vi "Make sine signal.vi"(0 "sinfreq":dbl, 1 "stimdur":dbl, 2 "nsamp":dbl, 3 "sinamp":dbl, 5 "Output freq (Hz)":dbl, 7 "hicutoff":dbl, 9 "lowcutoff":dbl, 11 "noiseamp":dbl, 12 "beforedur":dbl, 13 "afterdur":dbl) -> (4 "Stimulus out":T2 {"noise freq hi" min=0.0 step=0.5; "noise freq lo" min=0.0 step=0.5; "noiseamp end" min=0.0 step=0.5; "noiseamp start" min=0.0 step=0.5}, 6 "sine wave":dbl[](array[numeric]), 8 "noise":dbl[](array[numeric]), 10 "phases":T1)   [LabVIEW 2013]
uses:
  Stimulus.ctl
  Stimulus type.ctl
  Pulse data.ctl
  Phases.ctl
  <vilib>/Analysis/NI_AALBase.lvlib
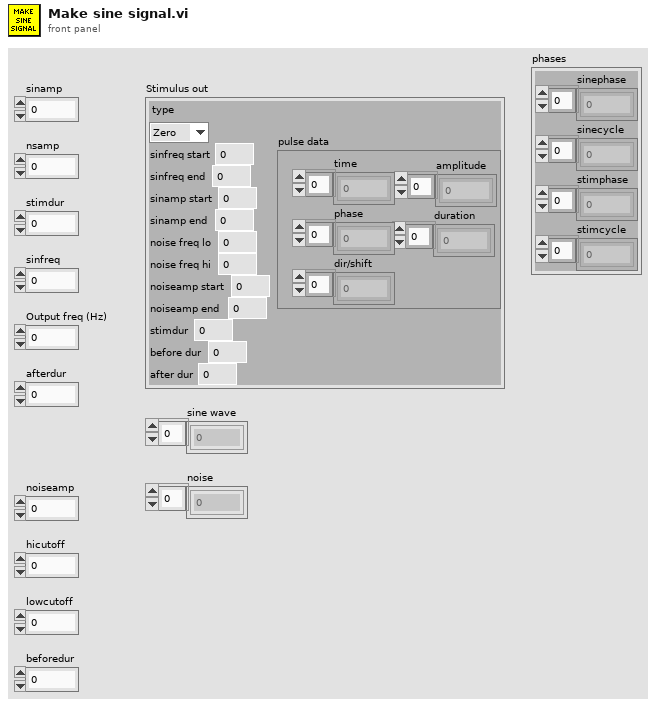
[diagram p1: front panel]
types:
  T1 = typedef "Phases.ctl" = cluster{"sinephase":dbl[], "sinecycle":dbl[], "stimphase":dbl[], "stimcycle":dbl[]}
  T2 = typedef "Stimulus.ctl" = cluster{"type":T3, "sinfreq start":dbl, "sinfreq end":dbl, "sinamp start":dbl, "sinamp end":dbl, "noise freq lo":dbl, "noise freq hi":dbl, "noiseamp start":dbl, "noiseamp end":dbl, "stimdur":dbl, "before dur":dbl, "after dur":dbl, "pulse data":T4}
  T3 = typedef "Stimulus type.ctl" = enum16{"Zero", "Sine", "Frequency sweep", "Two frequency", "Amplitude sweep", "Pulses", "Shifts"}
  T4 = typedef "Pulse data.ctl" = cluster{"time":dbl[], "phase":dbl[], "dir/shift":dbl[], "amplitude":dbl[], "duration":dbl[]}
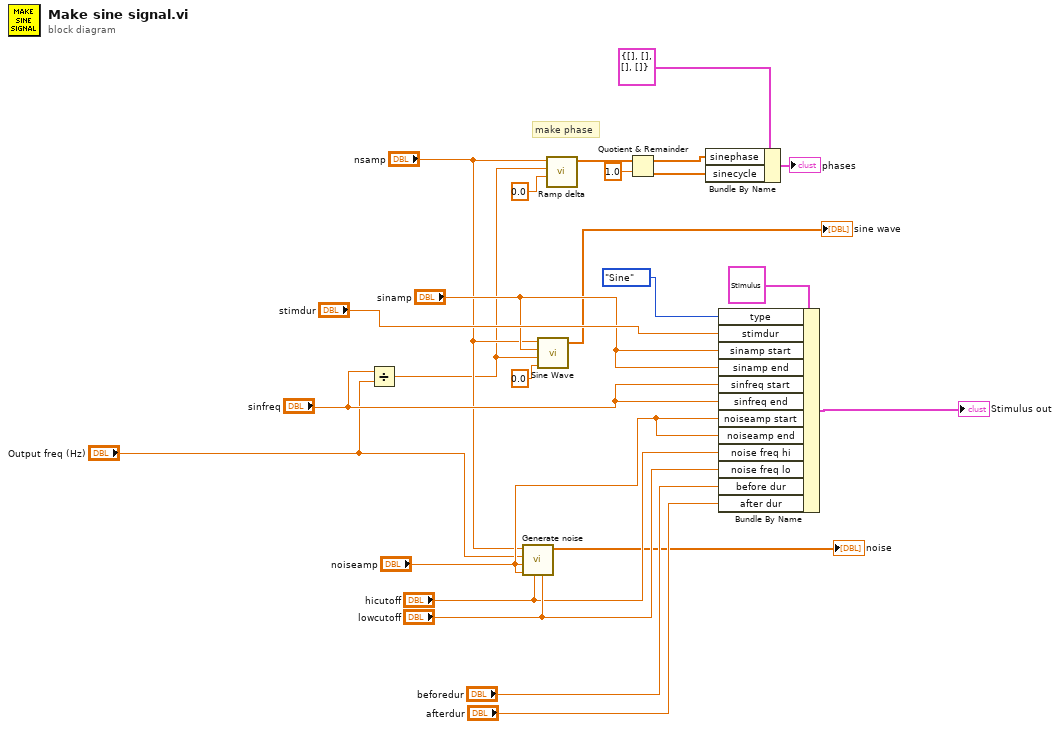
[diagram p0: block diagram]
diagram:
  # "make phase"
  n1 = Divide(x="sinfreq", y="Output freq (Hz)") -> (x/y=w8:dbl)
  n2 = call "Generate noise.vi"("lo cutoff"="lowcutoff", "hi cutoff"="hicutoff", "start amplitude"="noiseamp", "end amplitude"="noiseamp", "sampling freq"="Output freq (Hz)", "samples"="nsamp") -> ("noise"=→"noise":dbl[])  [unwired: 5 in]
  n3 = call <vilib>:"Sine Wave.vi"("samples"="nsamp", "amplitude"="sinamp", "frequency"=w8, "phase in"=0.0) -> ("sine wave"=→"sine wave":dbl[])  [unwired: 1 in, 2 out]
  n4 = call "Ramp delta.vi"("start"=0.0, "delta"=w8, "samples"="nsamp") -> ("ramp signal"=w6:dbl[])  [unwired: 7 in, 1 out]
  n5 = Quotient & Remainder(x=w6, y=1.0 ("start")) -> (x-y*floor(x/y)=w3:dbl[], floor(x/y)=w2:dbl[])
  n6 = Bundle By Name(cluster=T1 {"sinephase"=[], "sinecycle"=[], "stimphase"=[], "stimcycle"=[]} ("phases"), "sinephase"=w3, "sinecycle"=w2) -> (→"phases":T1)
  n7 = Bundle By Name(cluster=T2 {"type"=enum."Zero", "sinfreq start"=0.0, "sinfreq end"=0.0, "sinamp start"=0.0, "sinamp end"=0.0, "noise freq lo"=0.0, "noise freq hi"=0.0, "noiseamp start"=0.0, "noiseamp end"=0.0, "stimdur"=0.0, "before dur"=0.0, "after dur"=0.0, "pulse data"={"time"=[], "phase"=[], "dir/shift"=[], "amplitude"=[], "duration"=[]}} ("Stimulus 2"), "type"=Stimulus_type."Sine", "stimdur"="stimdur", "sinamp start"="sinamp", "sinamp end"="sinamp", "sinfreq start"="sinfreq", "sinfreq end"="sinfreq", "noiseamp start"="noiseamp", "noiseamp end"="noiseamp", "noise freq hi"="hicutoff", "noise freq lo"="lowcutoff", "before dur"="beforedur", "after dur"="afterdur") -> (→"Stimulus out":T2)
